vi "Actor Core.vi"(8 "error in":errorcluster, 11 "Composite User Interface in":refnum<class "Composite User Interface.lvclass">) -> (0 "error out":errorcluster, 3 "Actor out":refnum<class "Actor.lvclass">)   [LabVIEW 2017, in "2. Basic Panel Actors.lvlib" / "Composite User Interface.lvclass"]
doc: "The user interface for this panel.\n----\nCopyright: MGI 2016\nAuthor: Derek Trepanier"
uses:
  Composite User Interface.lvclass
  panel-manager/Source/MGI-Panel Manager.lvlib
  panel-manager/Source/Panel/Subpanel/Subpanel.vi
  panel-manager/Source/Panel/Subpanel/Subpanel.lvclass
  Description Panel/Description Panel.lvclass
  panel-actors/Source/Panel Actor/Panel Actor.lvclass
  <vilib>/ActorFramework/Stop Msg/Stop Msg.lvclass
  Data Manager/Data Manager.lvclass
  Data Viewer/Data Viewer.lvclass
  panel-manager/Source/Panel/Panel.lvclass
  D:/test/LabView_PanelManager/panel-manager/Source/Panel/Panel.lvclass
  D:/test/LabView_PanelManager/panel-actors/Source/Panel Actor/Panel Actor.lvclass
  <vilib>/ActorFramework/Actor/Actor.lvclass
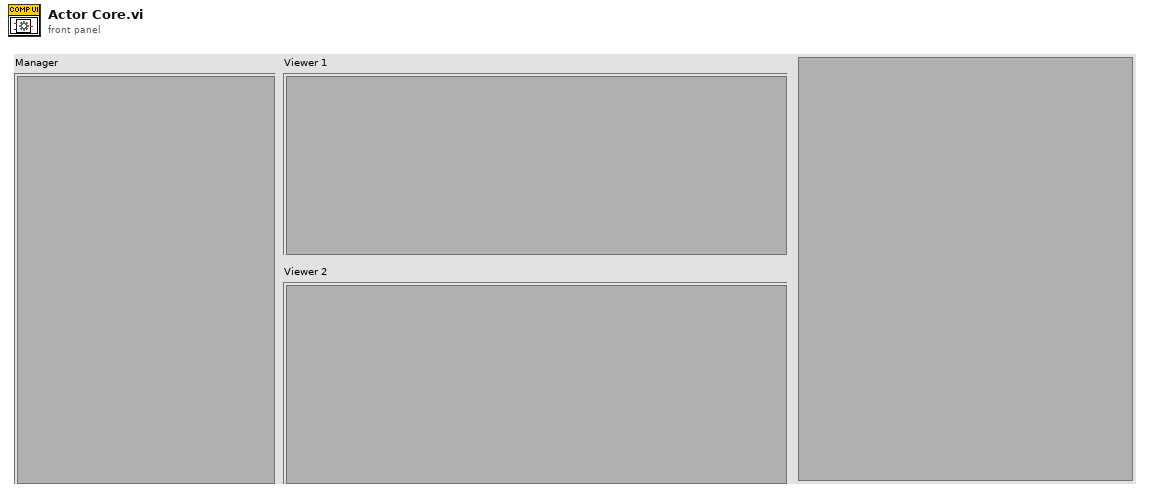
[diagram p1: front panel]
types:
  T1 = cluster{"Panel Actor":refnum<class "Panel Actor.lvclass">, "Panel":refnum<class "Panel.lvclass">}
  T2 = cluster{"Panel Actor":refnum<class "Panel Actor.lvclass">, "Panel":refnum<class "Panel.lvclass">}[]
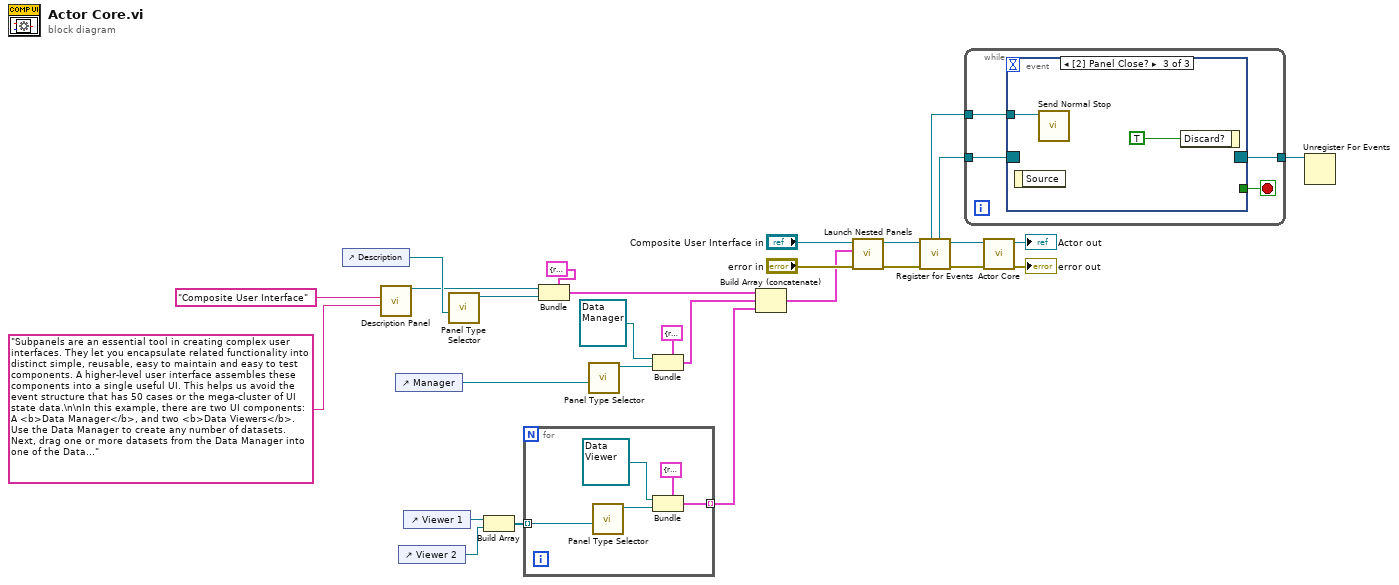
[diagram p0: block diagram]
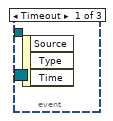
[diagram p2: hidden frame]
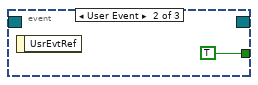
[diagram p3: hidden frame]
diagram:
  n1 = control-ref of="Description"() -> (w22:refnum<vi>)
  n2 = call "Description Panel.vi"("Description"="Subpanels are an essential tool in creating complex user interfaces. They let you encapsulate related functionality into distinct simple, reusable, easy to maintain and easy to test components. A higher-level user interface assembles these components into a single useful UI. This helps us avoid the event structure that has 50 cases or the mega-cluster of UI state data.\n\nIn this example, there are two UI components: A <b>Data Manager</b>, and two <b>Data Viewers</b>. Use the Data Manager to create any number of datasets. Next, drag one or more datasets from the Data Manager into one of the Data Viewers. \n\nNotice how the top-level UI is trivial. All it does is launch the components and manage closing the application. We also get some nice re-use with Data Viewer component by launching two of the same component in different subpanels on the top-level UI and by being able to launch a Dataset Viewer in a separate window from the Dataset Manager. \n" ("Description Title"), "Description Title"="Composite User Interface") -> ("Description Panel out"=w9:refnum<class "Description Panel.lvclass">)  [unwired: 8 in, 1 out]
  n3 = control-ref of="Manager"() -> (w19:refnum<vi>)
  n4 = control-ref of="Viewer 2"() -> (w17:refnum<vi>)
  n5 = control-ref of="Viewer 1"() -> (w18:refnum<vi>)
  n6 = call-poly "Panel Type Selector.vi"("Sub Panel"=w22) -> ("Subpanel Out"=w6:refnum<class "Subpanel.lvclass">)  [unwired: 9 in, 1 out]
  n7 = Build Array(w18, w17) -> (w16:refnum<vi>[])
  n8 = for {
    tunnel: w16 -> [w33] mode=indexing
    tunnel: [w30] -> w1 mode=indexing
    n9 = call-poly "Panel Type Selector.vi"("Sub Panel"=w33) -> ("Subpanel Out"=w32:refnum<class "Subpanel.lvclass">)  [unwired: 9 in, 1 out]
    n10 = Bundle(cluster=T1 {"Panel Actor"=refnum, "Panel"=refnum} ("Elements"), "Panel Actor"=refnum<class "Data Viewer.lvclass"> refnum ("2. Basic Panel Actors.lvlib:Data Viewer.lvclass"), "Panel"=w32) -> (w30:T1)
  }
  n11 = Bundle(cluster=T1 {"Panel Actor"=refnum, "Panel"=refnum} ("Elements"), "Panel Actor"=w9, "Panel"=w6) -> (w8:T1)
  n12 = call-poly "Panel Type Selector.vi"("Sub Panel"=w19) -> ("Subpanel Out"=w11:refnum<class "Subpanel.lvclass">)  [unwired: 9 in, 1 out]
  n13 = Bundle(cluster=T1 {"Panel Actor"=refnum, "Panel"=refnum} ("Elements"), "Panel Actor"=refnum<class "Data Manager.lvclass"> refnum ("2. Basic Panel Actors.lvlib:Data Manager.lvclass"), "Panel"=w11) -> (w7:T1)
  n14 = Build Array (concatenate)(w8, w7, w1) -> (w2:T2)
  n15 = call "Launch Nested Panels.vi"("error in (no error)"="error in", "Nested Panel Actors"=w2, "Panel Actor in"="Composite User Interface in") -> ("error out"=w14:errorcluster, "Panel Actor out"=w13:refnum<class "Composite User Interface.lvclass">)  [unwired: 5 in, 2 out]
  n16 = call "Register for Events.vi"("Error In"=w14, "Panel Actor in"=w13) -> ("Error Out"=w24:errorcluster, "Panel Actor out"=w23:refnum<class "Composite User Interface.lvclass">, "Pnl Actor"=w21:refnum<event-registration>, "Self Enqueuer"=w20:refnum<class "Message Enqueuer.lvclass">)  [unwired: 5 in, 1 out]
  n17 = while {
    tunnel: w21 -> [w37]
    tunnel: w20 -> [w36]
    tunnel: [w34] -> w15
    stop <- w35 stop-if-true
    n18 = event shown="[2] Panel Close?" {
      selector: w37 -> [_ _ _]
      dyn-events: [_ _ _] -> w34
      timeout: _ -> [_ _ _]
      tunnel: w36 -> [_ _ w40]
      tunnel: [_ TRUE _] -> w35
      event Timeout {
        n19 = event-data() -> ()  [unwired: 1 in, 3 out]
      }
      event User Event {
        n20 = event-data() -> ()  [unwired: 1 in, 1 out]
      }
      event Panel Close? {
        n21 = event-data() -> ()  [unwired: 1 in, 1 out]
        n22 = call <vilib>:"Send Normal Stop.vi"("Message Enqueuer"=w40) -> ()  [unwired: 10 in, 1 out]
        n23 = event-data("Discard?"=TRUE) -> ()  [unwired: 1 in, 1 out]
      }
    }
  }
  n24 = call-parent "Actor Core.vi"("error in"=w24, "Panel Actor in"=w23) -> ("error out"=→"error out":errorcluster, "Actor out"=→"Actor out":refnum<class "Actor.lvclass">)  [unwired: 8 in]
  n25 = Unregister For Events(event registration refnum=w15) -> ()  [unwired: 1 in, 1 out]
